vi "Find Closest Direction (Bob).vi"(11 "Bot Angle":dbl) -> (3 "Numeric":dbl)   [LabVIEW 2017]
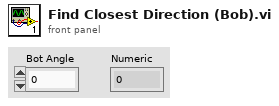
[diagram p1: front panel]
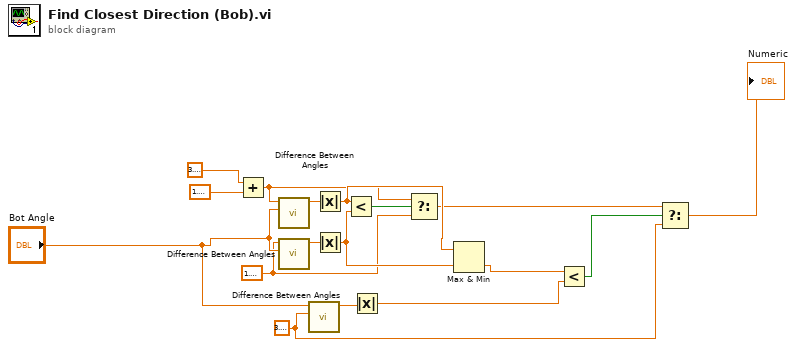
[diagram p0: block diagram]
diagram:
  w14 = 3.141592653589793
  w7 = 1.5707963267948966
  n1 = Add(x=3.141592653589793, y=1.5707963267948966) -> (x+y=w6:dbl)
  n2 = call "Difference Between Angles.vi"("Angle 2"="Bot Angle", "Angle 1"=w6) -> ("Difference"=w3:dbl)  [unwired: 9 in]
  n3 = call "Difference Between Angles.vi"("Angle 2"="Bot Angle", "Angle 1"=w7) -> ("Difference"=w4:dbl)  [unwired: 9 in]
  n4 = call "Difference Between Angles.vi"("Angle 2"=w14, "Angle 1"="Bot Angle") -> ("Difference"=w11:dbl)  [unwired: 9 in]
  n5 = Absolute Value(x=w3) -> (abs(x)=w9:dbl)
  n6 = Absolute Value(x=w4) -> (abs(x)=w10:dbl)
  n7 = Less?(x=w9, y=w10) -> (x < y?=w5:bool)
  n8 = Absolute Value(x=w11) -> (abs(x)=w12:dbl)
  n9 = Select(t=w6, s=w5, f=w7) -> (s? t:f=w8:dbl)
  n10 = Max & Min(x=w9, y=w10) -> (min(x,y)=w16:dbl)  [unwired: 1 out]
  n11 = Less?(x=w16, y=w12) -> (x < y?=w13:bool)
  n12 = Select(t=w8, s=w13, f=w14) -> (s? t:f=→"Numeric":dbl)
